vi "Stanford Research 844 Fast Mode Measurement.vi"(0 "VISA Resource Name":refnum<visa-resource-name>="GPIB0::8::INSTR", 2 "Data Sample Rate (10: 64 Hz)":u16(ring)=10 items=["62.5 mHz", "125 mHz", "250 mHz", "500 mHz", "1 Hz", "2 Hz", "4 Hz", "8 Hz", "16 Hz", "32 Hz", "64 Hz", "128 Hz", "256 Hz", "512 Hz", "Trigger"], 3 "Number Of Points (64)":u32=64) -> (17 "Array of X":dbl[](array[numeric]) format="%.2p", 18 "Array of  Y":dbl[](array[numeric]) format="%.2p")   [LabVIEW 2010]
doc: "This VI shows how to use fast data transfer mode.\n\nImportant: This VI is for GPIB only."
uses:
  <instrlib>/Stanford Research 844/Stanford Research 844.lvlib
panel:
  # "© 2005 National Instruments.  ALL RIGHTS RESERVED."
  # "GPIB only !!!"
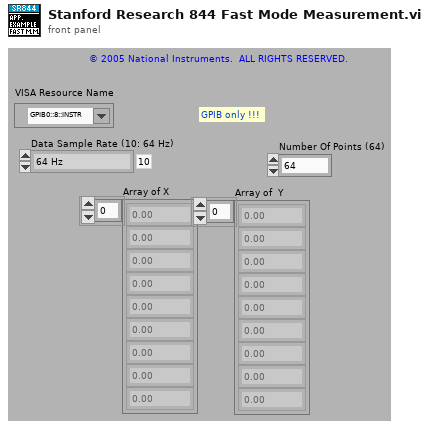
[diagram p1: front panel]
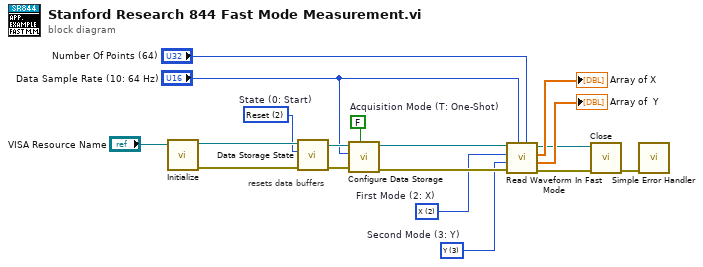
[diagram p0: block diagram]
diagram:
  w6 = u16 3 items=["R [V]", "Theta", "X", "Y"]  # Second Mode (3: Y)
  w7 = u16 2 items=["R [V]", "Theta", "X", "Y"]  # First Mode (2: X)
  w8 = FALSE  # Acquisition Mode (T: One-Shot)
  w17 = u16 2 items=["Start", "Pause", "Reset"]  # State (0: Start)
  # "resets data buffers"
  n1 = call <instrlib>:"Initialize.vi"("VISA Resource Name"="VISA Resource Name") -> ("error out"=w1:errorcluster, "VISA Resource Name Out"=w18:refnum<visa-resource-name>)  [unwired: 9 in]
  n2 = call <instrlib>:"Data Storage State.vi"("Error In (no error)"=w1, "State (0: Start)"=w17, "VISA Resource Name"=w18) -> ("Error Out"=w15:errorcluster, "VISA Resource Name Out"=w16:refnum<visa-resource-name>)  [unwired: 7 in]
  n3 = call <instrlib>:"Configure Data Storage.vi"("Acquisition Mode (T: One-Shot)"=w8, "Error In (no error)"=w15, "Data Sample Rate (0: 62.5 mHz)"="Data Sample Rate (10: 64 Hz)", "VISA Resource Name"=w16) -> ("Error Out"=w9:errorcluster, "VISA Resource Name Out"=w10:refnum<visa-resource-name>)  [unwired: 6 in]
  n4 = call <instrlib>:"Read Waveform In Fast Mode.vi"("Number Of Points (64)"="Number Of Points (64)", "Data Sample Rate (0: 62.5 mHz)"="Data Sample Rate (10: 64 Hz)", "Error In (no error)"=w9, "Second Output Mode (3: Y)"=w6, "First Output Mode (2: X)"=w7, "VISA Resource Name"=w10) -> ("Error Out"=w4:errorcluster, "Second Output Mode Array"=→"Array of  Y":dbl[], "First Output Mode Array"=→"Array of X":dbl[], "VISA Resource Name Out"=w5:refnum<visa-resource-name>)  [unwired: 2 in]
  n5 = call <instrlib>:"Close.vi"("error in (no error)"=w4, "VISA Resource Name"=w5) -> ("error out"=w3:errorcluster)  [unwired: 9 in]
  n6 = call <vilib>:"Simple Error Handler.vi"("error in (no error)"=w3) -> ()  [unwired: 4 in, 5 out]
